vi "update_run_mode.vi"(8 "error in (no error)":errorcluster, 11 "DL090202ScanHead in":refnum<class "ScanHeadDL090202.lvclass">) -> (0 "error out":errorcluster, 3 "DL090202ScanHead out":refnum<class "ScanHeadDL090202.lvclass">)   [LabVIEW 2010, in "ScanHeadDL090202.lvclass"]
uses:
  ScanHeadDL090202.lvclass
  Trajectory/TrajectoryDL091126GenericVoxel/TrajectoryDL091126GenericVoxel/TrajectoryDL091126GenericVoxel.lvclass
  Clock/GenericClock/GenericClock/GenericClock.lvclass
  DAQ/GenericDAQ/GenericDAQ/GenericDAQ.lvclass
  SignalWriter/GenericSignalWriter/GenericSignalWriter/GenericSignalWriter.lvclass
  common/classes/ErrorController/ErrorController/class_data.vi
  common/classes/ErrorController/ErrorController/ErrorController.lvclass
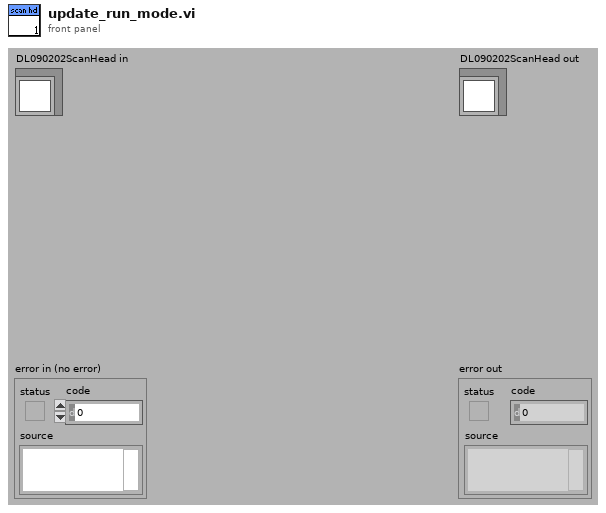
[diagram p1: front panel]
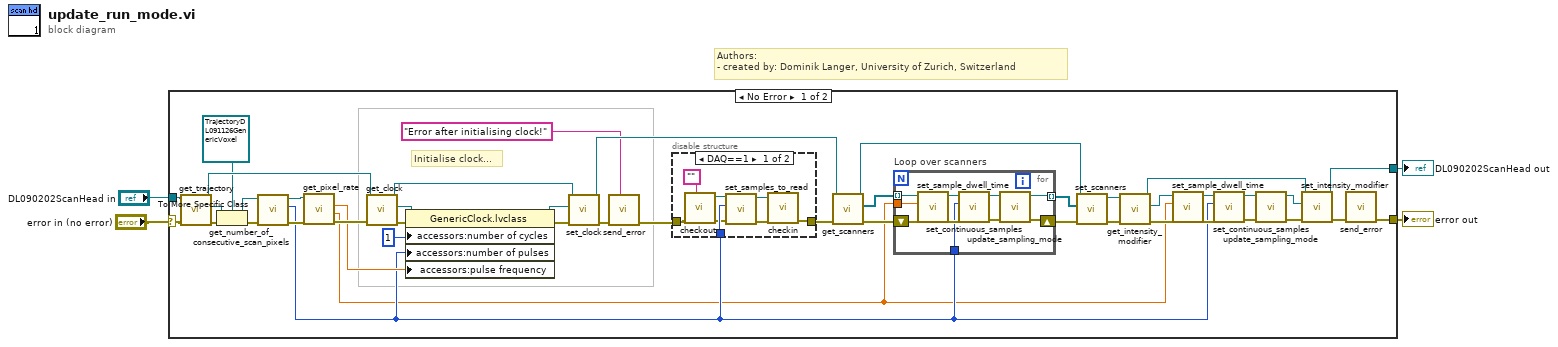
[diagram p0: block diagram]
diagram:
  # "Authors: \n- created by: Dominik Langer, University of Zurich, Switzerland"
  n1 = case shown="No Error" "error in (no error)" {
    selector: "error in (no error)" -> [w10 w69]
    tunnel: [w15 w69] -> w3
    tunnel: [w48 w68] -> w1
    tunnel: "DL090202ScanHead in" -> [w9 w68]
    frame No Error {
      # "Initialise clock..."
      n2 = call-dynamic "get_trajectory.vi"("error in (no error)"=w10, "GenericScanHead.lvclass in"=w9) -> ("error out"=w31:errorcluster, "trajectory"=w28:refnum<class "GenericTrajectory.lvclass">, "GenericScanHead.lvclass out"=w46:refnum<class "ScanHeadDL090202.lvclass">)  [unwired: 7 out]
      n3 = To More Specific Class(target class=refnum<class "TrajectoryDL091126GenericVoxel.lvclass"> refnum ("TrajectoryDL091126GenericVoxel.lvclass"), reference=w28, error in=w31) -> (specific class reference=w27:refnum<class "TrajectoryDL091126GenericVoxel.lvclass">, error out=w30:errorcluster)
      n4 = call-dynamic "get_number_of_consecutive_scan_pixels.vi"("error in (no error)"=w30, "GenericTrajectory in"=w27) -> ("error out"=w22:errorcluster, "number of consecutive scan pixels"=w6:i64, "GenericTrajectory out"=w21:refnum<class "TrajectoryDL091126GenericVoxel.lvclass">)  [unwired: 7 out]
      n5 = call-dynamic "get_pixel_rate.vi"("error in (no error)"=w22, "GenericTrajectory in"=w21) -> ("error out"=w20:errorcluster, "pixel dwell time"=w5:dbl[unit], "pixel rate"=w7:dbl[unit])  [unwired: 6 in, 1 out]
      n6 = call-dynamic "get_clock.vi"("error in (no error)"=w20, "DL090202ScanHead.lvclass in"=w46) -> ("error out"=w12:errorcluster, "GenericClock.lvclass"=w13:refnum<class "GenericClock.lvclass">, "DL090202ScanHead.lvclass out"=w47:refnum<class "ScanHeadDL090202.lvclass">)  [unwired: 7 out]
      n7 = property class="GenericClock.lvclass"(reference=w13, error in=w12, "accessors:number of cycles"=i64 1 ("number of cycles"), "accessors:number of pulses"=w6, "accessors:pulse frequency"=w7) -> (reference out=w14:refnum<class "GenericClock.lvclass">, error out=w11:errorcluster)
      n8 = call-dynamic "set_clock.vi"("error in (no error)"=w11, "GenericClock.lvclass"=w14, "DL090202ScanHead.lvclass in"=w47) -> ("error out"=w19:errorcluster, "DL090202ScanHead.lvclass out"=w44:refnum<class "ScanHeadDL090202.lvclass">)  [unwired: 7 out]
      n9 = call "send_error.vi"("additional message"="Error after initialising clock!", "error in (no error)"=w19) -> ("error out"=w18:errorcluster)  [unwired: 9 in]
      n10 = disable-structure shown="DAQ==1" {
        disable-tunnel: [w62 w67] -> w45
        disable-tunnel: w18 -> [w65 w67]
        disable-tunnel: w6 -> [w66 _]
        frame condition #0 (active) {
          n11 = call "checkout.vi"("locked by?"="", "error in (no error)"=w65) -> ("error out"=w64:errorcluster, "GenericDAQ out"=w60:refnum<class "GenericDAQ.lvclass">)  [unwired: 8 in]
          n12 = call-dynamic "set_samples_to_read.vi"("error in (no error)"=w64, "samples to read"=w66, "GenericDAQ.lvclass in"=w60) -> ("error out"=w63:errorcluster, "GenericDAQ.lvclass out"=w59:refnum<class "GenericDAQ.lvclass">)  [unwired: 7 out]
          n13 = call-dynamic "checkin.vi"("error in (no error)"=w63, "GenericDAQ in"=w59) -> ("error out"=w62:errorcluster)  [unwired: 8 in, 1 out]
        }
        frame condition #1 {
        }
      }
      n14 = call-dynamic "get_scanners.vi"("error in (no error)"=w45, "DL090202ScanHead.lvclass in"=w44) -> ("error out"=w43:errorcluster, "scanners"=w42:refnum<class "GenericSignalWriter.lvclass">[], "DL090202ScanHead.lvclass out"=w39:refnum<class "ScanHeadDL090202.lvclass">)  [unwired: 7 out]
      n15 = for "Loop over scanners" {
        shift-right: [w57] -> w40
        shift-left: w43 -> [w56]
        tunnel: w42 -> [w54] mode=indexing
        tunnel: [w58] -> w36 mode=indexing
        tunnel: w6 -> [w51]
        tunnel: w5 -> [w52]
        n16 = call-dynamic "set_sample_dwell_time.vi"("error in (no error)"=w56, "sample dwell time"=w52, "GenericWriteSignals.lvclass in"=w54) -> ("error out"=w55:errorcluster, "GenericWriteSignals.lvclass out"=w53:refnum<class "GenericSignalWriter.lvclass">)  [unwired: 7 out]
        n17 = call-dynamic "set_continuous_samples.vi"("error in (no error)"=w55, "continuous samples"=w51, "GenericWriteSignals.lvclass in"=w53) -> ("error out"=w50:errorcluster, "GenericWriteSignals.lvclass out"=w49:refnum<class "GenericSignalWriter.lvclass">)  [unwired: 7 out]
        n18 = call-dynamic "update_sampling_mode.vi"("error in (no error)"=w50, "GenericWriteSignals in"=w49) -> ("error out"=w57:errorcluster, "GenericWriteSignals out"=w58:refnum<class "GenericSignalWriter.lvclass">)  [unwired: 8 out]
      }
      n19 = call-dynamic "set_scanners.vi"("error in (no error)"=w40, "scanners"=w36, "DL090202ScanHead.lvclass in"=w39) -> ("error out"=w41:errorcluster, "DL090202ScanHead.lvclass out"=w38:refnum<class "ScanHeadDL090202.lvclass">)  [unwired: 7 out]
      n20 = call-dynamic "get_intensity_modifier.vi"("error in (no error)"=w41, "DL090202ScanHead.lvclass in"=w38) -> ("error out"=w35:errorcluster, "write signals"=w33:refnum<class "GenericSignalWriter.lvclass">, "DL090202ScanHead.lvclass out"=w37:refnum<class "ScanHeadDL090202.lvclass">)  [unwired: 7 out]
      n21 = call-dynamic "set_sample_dwell_time.vi"("error in (no error)"=w35, "sample dwell time"=w5, "GenericWriteSignals.lvclass in"=w33) -> ("error out"=w26:errorcluster, "GenericWriteSignals.lvclass out"=w25:refnum<class "GenericSignalWriter.lvclass">)  [unwired: 7 out]
      n22 = call-dynamic "set_continuous_samples.vi"("error in (no error)"=w26, "continuous samples"=w6, "GenericWriteSignals.lvclass in"=w25) -> ("error out"=w24:errorcluster, "GenericWriteSignals.lvclass out"=w23:refnum<class "GenericSignalWriter.lvclass">)  [unwired: 7 out]
      n23 = call-dynamic "update_sampling_mode.vi"("error in (no error)"=w24, "GenericWriteSignals in"=w23) -> ("error out"=w34:errorcluster, "GenericWriteSignals out"=w32:refnum<class "GenericSignalWriter.lvclass">)  [unwired: 8 out]
      n24 = call-dynamic "set_intensity_modifier.vi"("error in (no error)"=w34, "write signals"=w32, "DL090202ScanHead.lvclass in"=w37) -> ("error out"=w16:errorcluster, "DL090202ScanHead.lvclass out"=w48:refnum<class "ScanHeadDL090202.lvclass">)  [unwired: 7 out]
      n25 = call "send_error.vi"("error in (no error)"=w16) -> ("error out"=w15:errorcluster)  [unwired: 10 in]
    }
    frame Error {
    }
  }
  "error out" <- w3
  "DL090202ScanHead out" <- w1
